vi "SP Enqueue Element.vi"(8 "error in (no error)":errorcluster, 9 "Timeout In (ms)":i32=100, 10 "Queue Cluster":T1={"Command"="", "Test Parameters"={"Stimulus"={"Use Instrument Settings"=FALSE, "Blank Frequencies"=FALSE, "Sweep Type"=enum."Linear", "Sweep"={"Fstart"=500.0, "Fstop"=1500.0, "Units"=enum."MHz", "Points"=2}, "Power (dBm)"=999.0, "IFBW (Hz)"=-1.0, "Sweep Time (s)"=-1.0, "Calibration"={"State"=FALSE, "String"=""}}, "Measurement"={"Auto Select"=TRUE, "Data Source"=enum."VNA", "Ports"=2, "Parameters"=[]}, "De-Embed"={"De-Embed"=FALSE, "Adapters"=[]}, "Display"={"Lock Control"=FALSE, "Retain Settings"=TRUE, "Formatted Data"=FALSE, "Plot Orientation"=enum."Single", "Plot Controls"=[{"Trace Orientation"=enum."Overlay", "Frequency"={"Change Frequency"=FALSE, "Start"=500.0, "Stop"=1500.0, "Units"=enum."MHz"}, "Markers"=[], "Traces"=[]}, {"Trace Orientation"=enum."Overlay", "Frequency"={"Change Frequency"=FALSE, "Start"=500.0, "Stop"=1500.0, "Units"=enum."MHz"}, "Markers"=[], "Traces"=[]}, {"Trace Orientation"=enum."Overlay", "Frequency"={"Change Frequency"=FALSE, "Start"=500.0, "Stop"=1500.0, "Units"=enum."MHz"}, "Markers"=[], "Traces"=[]}, {"Trace Orientation"=enum."Overlay", "Frequency"={"Change Frequency"=FALSE, "Start"=500.0, "Stop"=1500.0, "Units"=enum."MHz"}, "Markers"=[], "Traces"=[]}]}, "Limits"=[], "Filter Limits"=[]}} {"Test Parameters"."Filter Limits"."Parameter"."Stimulus Port" min=1 step=1; "Test Parameters"."Filter Limits"."Parameter"."Response Port" min=1 step=1; "Test Parameters"."Filter Limits"."Passband"."Bandwidth Attn" format="%.3g"; "Test Parameters"."Filter Limits"."Passband"."Stop/Span" format="%.3g"; "Test Parameters"."Filter Limits"."Passband"."Start/Center" format="%.3g"; "Test Parameters"."Measurement"."Parameters"."Channel" min=0 max=32 step=1; "Test Parameters"."Measurement"."Parameters"."Parameter"."Stimulus Port" min=1 step=1; "Test Parameters"."Measurement"."Parameters"."Parameter"."Response Port" min=1 step=1; "Test Parameters"."Limits"."Parameter"."Stimulus Port" min=1 step=1; "Test Parameters"."Limits"."Parameter"."Response Port" min=1 step=1; "Test Parameters"."Stimulus"."Sweep Time (s)" format="%.3g"; "Test Parameters"."Display"."Plot Controls"."Traces"."Reference" format="%#.2g"; "Test Parameters"."Display"."Plot Controls"."Traces"."Scale" min=0.001 step=1.0 format="%#.2g"; "Test Parameters"."Display"."Plot Controls"."Traces"."Position" min=0.0 max=10.0; "Test Parameters"."Display"."Plot Controls"."Frequency"."Stop" format="%.3g"; "Test Parameters"."Display"."Plot Controls"."Frequency"."Start" format="%.3g"}, 11 "Queue":refnum<queue>) -> (0 "error out":errorcluster, 1 "Timed Out?":bool, 3 "Queue":refnum<queue>)   [LabVIEW 2011]
uses:
  TypeDefs/SP Queue Cluster.ctl
  TypeDefs/SP Test Parameters.ctl
  TypeDefs/SP Stimulus Parameters.ctl
  TypeDefs/SP Frequency Units.ctl
  TypeDefs/SP Calibration State.ctl
  TypeDefs/SP Measurement.ctl
  TypeDefs/SP Parameters.ctl
  TypeDefs/SP Parameter.ctl
  TypeDefs/SP De-Embed.ctl
  TypeDefs/SP Adapter.ctl
  TypeDefs/SP Data.ctl
  TypeDefs/SP Display Parameters.ctl
  TypeDefs/SP Display Plot Controls Cluster.ctl
  TypeDefs/SP Marker Cluster.ctl
  TypeDefs/SP Marker Type.ctl
  TypeDefs/SP Display Trace Controls.ctl
  TypeDefs/SP Display Format.ctl
  TypeDefs/SP Display Data.ctl
  TypeDefs/SP Limit.ctl
  TypeDefs/SP Format.ctl
  TypeDefs/SP Limit Type.ctl
  TypeDefs/SP Limit Point.ctl
  Test Referential Limit.ctl
  TypeDefs/SP Filter.ctl
  TypeDefs/SP Filter Type.ctl
  TypeDefs/SP Filter Passband.ctl
  TypeDefs/SP Frequency Format.ctl
  TypeDefs/SP Filter Ripple.ctl
  TypeDefs/SP Attenuation Point.ctl
  TypeDefs/SP Attenuation Type.ctl
  TypeDefs/SP Skirt Rejection Point.ctl
  TypeDefs/SP Relative Loss.ctl
panel:
  # "Div"
  # "Div"
  # "Div"
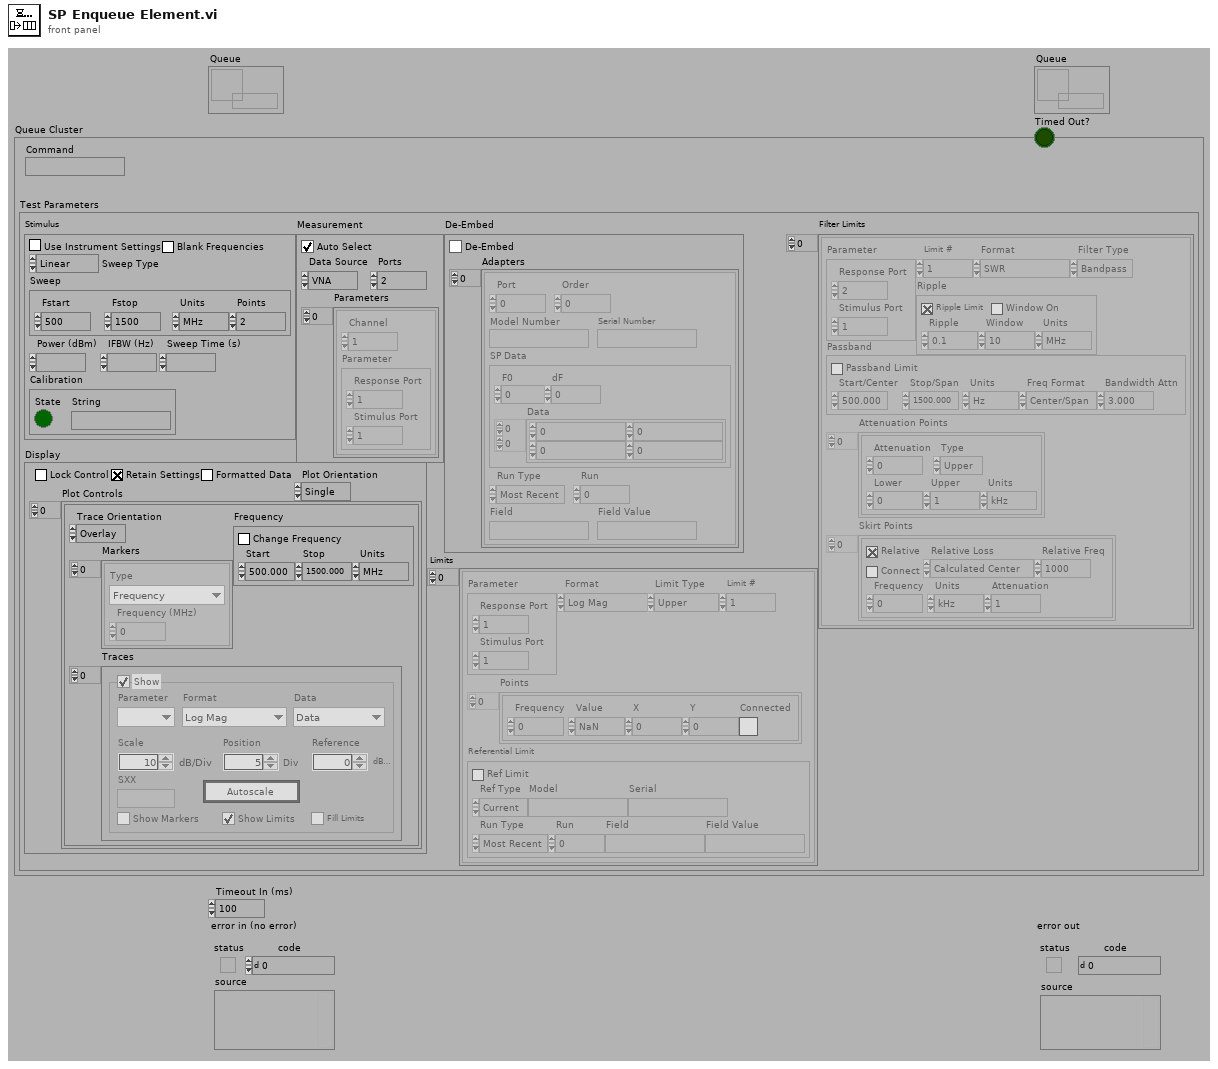
[diagram p1: front panel]
types:
  T1 = typedef "SP Queue Cluster.ctl" = cluster{"Command":string, "Test Parameters":T2}
  T2 = typedef "SP Test Parameters.ctl" = cluster{"Stimulus":T3, "Measurement":T6, "De-Embed":T9, "Display":T12, "Limits":T19[], "Filter Limits":T24[]}
  T3 = typedef "SP Stimulus Parameters.ctl" = cluster{"Use Instrument Settings":bool, "Blank Frequencies":bool, "Sweep Type":enum32{"Linear", "Logarithmic", "List", "Power", "CW"}, "Sweep":cluster{"Fstart":dbl, "Fstop":dbl, "Units":T4, "Points":i32}, "Power (dBm)":dbl, "IFBW (Hz)":dbl, "Sweep Time (s)":dbl, "Calibration":T5}
  T4 = typedef "SP Frequency Units.ctl" = enum16{"Hz", "kHz", "MHz", "GHz", "Points"}
  T5 = typedef "SP Calibration State.ctl" = cluster{"State":bool, "String":string}
  T6 = typedef "SP Measurement.ctl" = cluster{"Auto Select":bool, "Data Source":enum16{"VNA", "Data File"}, "Ports":i8, "Parameters":T7[]}
  T7 = typedef "SP Parameters.ctl" = cluster{"Channel":i8, "Parameter":T8}
  T8 = typedef "SP Parameter.ctl" = cluster{"Stimulus Port":i8, "Response Port":i8}
  T9 = typedef "SP De-Embed.ctl" = cluster{"De-Embed":bool, "Adapters":T10[]}
  T10 = typedef "SP Adapter.ctl" = cluster{"Port":i8, "Order":i8, "Model Number":string, "Serial Number":string, "SP Data":T11, "Run Type":enum16{"Most Recent", "Run #", "Match Field"}, "Run":i32, "Field":string, "Field Value":string}
  T11 = typedef "SP Data.ctl" = cluster{"F0":dbl, "dF":dbl, "Data":cdb[][]}
  T12 = typedef "SP Display Parameters.ctl" = cluster{"Lock Control":bool, "Retain Settings":bool, "Formatted Data":bool, "Plot Orientation":enum32{"Single", "Dual", "Quad"}, "Plot Controls":T13[]}
  T13 = typedef "SP Display Plot Controls Cluster.ctl" = cluster{"Trace Orientation":enum32{"Overlay", "Split"}, "Frequency":cluster{"Change Frequency":bool, "Start":dbl, "Stop":dbl, "Units":T4}, "Markers":T14[], "Traces":T16[]}
  T14 = typedef "SP Marker Cluster.ctl" = cluster{"Type":T15, "Frequency (MHz)":dbl}
  T15 = typedef "SP Marker Type.ctl" = enum16{"Frequency", "Trace Maximum", "Trace Minimum", "Limit Maximum", "Limit Minimum"}
  T16 = typedef "SP Display Trace Controls.ctl" = cluster{"Trace On":bool, "Measure":i32, "Format":T17, "Autoscale":bool, "Reference":dbl, "\nRefUnit":string, "Position":dbl, "Scale":dbl, "ScaleUnit":string, "LimitOn":bool, "LimitFill":bool, "Display Data":T18, "Show Markers":bool, "SXX":string}
  T17 = typedef "SP Display Format.ctl" = i32
  T18 = typedef "SP Display Data.ctl" = u16
  T19 = typedef "SP Limit.ctl" = cluster{"Parameter":T8, "Format":T20, "Limit Type":T21, "Points":T22[], "Referential Limit":T23, "Limit #":i8}
  T20 = typedef "SP Format.ctl" = enum16{"Log Mag", "Lin Mag", "SWR", "Phase", "Expanded Phase", "Delay", "Insertion Loss", "Isolation", "Return Loss"}
  T21 = typedef "SP Limit Type.ctl" = enum16{"Upper", "Lower", "Delta", "Filter", "Referential"}
  T22 = typedef "SP Limit Point.ctl" = cluster{"Frequency":dbl, "Value":dbl, "X":dbl, "Y":dbl, "Connected":bool}
  T23 = typedef "Test Referential Limit.ctl" = cluster{"Ref Limit":bool, "Ref Type":enum16{"Current", "Specify"}, "Model":string, "Serial":string, "Run Type":enum16{"Most Recent", "Run #", "Match Field"}, "Run":i32, "Field":string, "Field Value":string}
  T24 = typedef "SP Filter.ctl" = cluster{"Limit #":i8, "Parameter":T8, "Format":T20, "Filter Type":T25, "Passband":T26, "Ripple":T28, "Attenuation Points":T29[], "Skirt Points":T31[]}
  T25 = typedef "SP Filter Type.ctl" = enum16{"Lowpass", "Highpass", "Bandpass", "Bandstop"}
  T26 = typedef "SP Filter Passband.ctl" = cluster{"Start/Center":dbl, "Stop/Span":dbl, "Units":T4, "Freq Format":T27, "Bandwidth Attn":dbl, "Passband Limit":bool}
  T27 = typedef "SP Frequency Format.ctl" = enum16{"Start/Stop", "Center/Span"}
  T28 = typedef "SP Filter Ripple.ctl" = cluster{"Ripple Limit":bool, "Window On":bool, "Ripple":dbl, "Window":dbl, "Units":T4}
  T29 = typedef "SP Attenuation Point.ctl" = cluster{"Attenuation":dbl, "Type":T30, "Lower":dbl, "Upper":dbl, "Units":T4}
  T30 = typedef "SP Attenuation Type.ctl" = enum16{"Center", "Lower", "Upper"}
  T31 = typedef "SP Skirt Rejection Point.ctl" = cluster{"Relative":bool, "Connect":bool, "Frequency":dbl, "Units":T4, "Attenuation":dbl, "Relative Loss":T32, "Relative Freq":dbl}
  T32 = typedef "SP Relative Loss.ctl" = enum16{"Calculated Center", "Passband Minimum", "Passband Maximum", "Passband Average", "Frequency"}
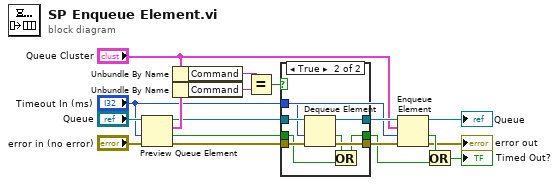
[diagram p0: block diagram]
diagram:
  n1 = Preview Queue Element(queue="Queue", timeout in ms (-1)="Timeout In (ms)", error in (no error)="error in (no error)") -> (queue out=w15:refnum<queue>, element=w16:T1, timed out?=w10:bool, error out=w11:errorcluster)
  n2 = Unbundle By Name("Queue Cluster") -> ("Command"=w13:string)
  n3 = Unbundle By Name(w16) -> ("Command"=w14:string)
  n4 = Equal?(x=w13, y=w14) -> (x = y?=w12:bool)
  n5 = case shown="True" w12 {
    tunnel: w15 -> [w21 w29]
    tunnel: w11 -> [w20 w28]
    tunnel: "Timeout In (ms)" -> [_ w27]
    tunnel: w10 -> [w19 w24]
    tunnel: [w20 w26] -> w9
    tunnel: [w21 w25] -> w8
    tunnel: [w19 w22] -> w5
    frame False {
    }
    frame True {
      n6 = Dequeue Element(queue=w29, timeout in ms (-1)=w27, error in (no error)=w28) -> (queue out=w25:refnum<queue>, timed out?=w23:bool, error out=w26:errorcluster)  [unwired: 1 out]
      n7 = Or(x=w23, y=w24) -> (x .or. y?=w22:bool)
    }
  }
  n8 = Enqueue Element(queue=w8, element="Queue Cluster", timeout in ms (-1)="Timeout In (ms)", error in (no error)=w9) -> (queue out=→"Queue":refnum<queue>, timed out?=w4:bool, error out=→"error out":errorcluster)
  n9 = Or(x=w4, y=w5) -> (x .or. y?=→"Timed Out?":bool)
